vi "Set Custom Device Initialization Time.vi"(8 "error in":errorcluster, 9 "Init Time":dbl format="%_19f", 10 "Execution.Settings":variant, 11 "VS Plugin API in":refnum<class "VS Custom Device API.lvclass">) -> (0 "error out":errorcluster, 3 "VS Plugin API out":refnum<class "VS Custom Device API.lvclass">)   [LabVIEW 2026, in "Template Engine.lvlib"]
uses:
  Template Engine.lvlib
  VS Custom Device API/VS Custom Device API.lvclass
  <vilib>/NI VeriStand/Custom Device API/Data Reference.ctl
  <vilib>/NI VeriStand/Custom Device API/Custom Device API.lvlib
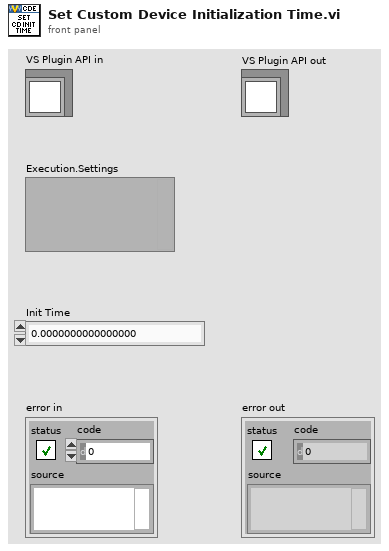
[diagram p1: front panel]
types:
  T1 = typedef "Custom Device API.lvlib/Data Reference.ctl" = i32
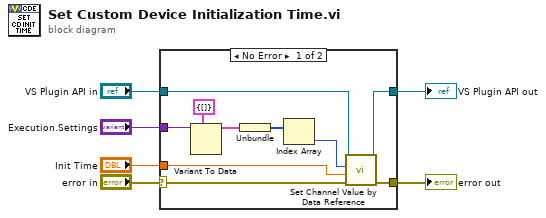
[diagram p0: block diagram]
diagram:
  n1 = case shown="No Error" "error in" {
    selector: "error in" -> [w8 w18]
    tunnel: "Execution.Settings" -> [w13 _]
    tunnel: [w16 w18] -> w5
    tunnel: "VS Plugin API in" -> [w7 w17]
    tunnel: "Init Time" -> [w11 _]
    tunnel: [w10 w17] -> w1
    frame No Error {
      n2 = Variant To Data(type=cluster{"Execution Channel Refs":T1[]} {"Execution Channel Refs"=[]}, Variant=w13) -> (data=w14:cluster{"Execution Channel Refs":T1[]})  [unwired: 1 in, 1 out]
      n3 = Unbundle(w14) -> ("Execution Channel Refs"=w12:T1[])
      n4 = Index Array(array=w12) -> (element=w9:T1)  [unwired: 1 in]
      n5 = call-dynamic "Set Channel Value by Data Reference.vi"("error in"=w8, "Value"=w11, "Data Reference in"=w9, "VS CDAPI in"=w7) -> ("error out"=w16:errorcluster, "VS CDAPI out"=w10:refnum<class "VS Custom Device API.lvclass">)  [unwired: 6 in]
    }
    frame Error {
    }
  }
  "error out" <- w5
  "VS Plugin API out" <- w1
